vi "strip returns.vi"(8 "error in (no error)":errorcluster, 11 "Language data":T1) -> (0 "error out":errorcluster, 3 "Language data out":T1)   [LabVIEW 2015, in "AguaClara Library.lvlib"]
uses:
  AguaClara Library.lvlib
  Variable cluster.ctl
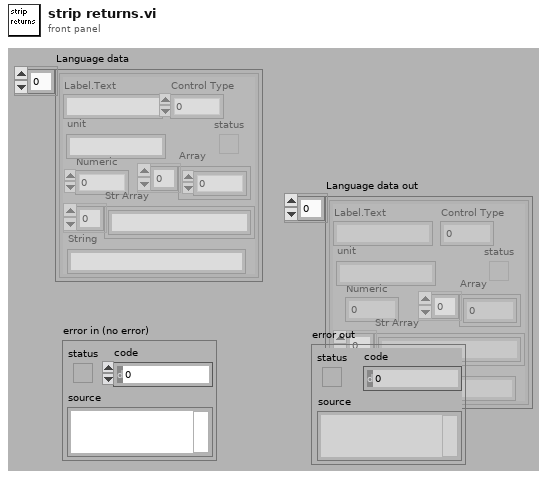
[diagram p1: front panel]
types:
  T1 = typedef "Variable cluster.ctl" = cluster{"Label.Text":string, "Control Type":u32, "Numeric":dbl, "Array":dbl[], "status":bool, "Str Array":string[], "String":string, "unit":string}[]
  T2 = cluster{"Label.Text":string, "Control Type":u32, "Numeric":dbl, "Array":dbl[], "status":bool, "Str Array":string[], "String":string, "unit":string}
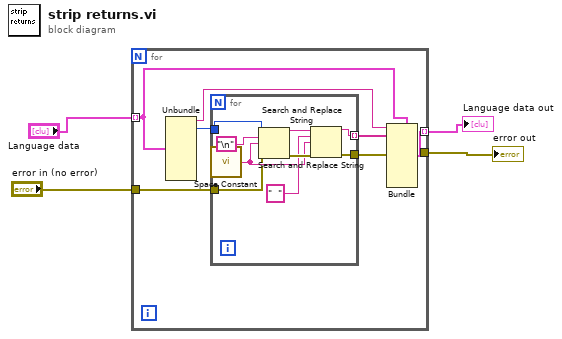
[diagram p0: block diagram]
diagram:
  n1 = for {
    tunnel: "Language data" -> [w10] mode=indexing
    tunnel: [w7] -> w3 mode=indexing
    tunnel: "error in (no error)" -> [w6]
    tunnel: [w5] -> w1
    n2 = Unbundle(w10) -> ("Label.Text"=w9:string, "Control Type"=w11:u32)  [unwired: 6 out]
    n3 = for {
      tunnel: w11 -> [w20]
      tunnel: [w15] -> w8 mode=indexing
      tunnel: w6 -> [w14]
      tunnel: [w13] -> w5
      n4 = call <vilib>:"Space Constant.vi"() -> ("String"=w16:string)
      n5 = Search and Replace String(input string=w20, search string="\n", replace string=w16, error in=w14) -> (result string=w19:string, error out=w18:errorcluster)  [unwired: 4 in, 2 out]
      n6 = Search and Replace String(input string=w19, search string="  ", replace string=w16, error in=w18) -> (result string=w15:string, error out=w13:errorcluster)  [unwired: 4 in, 2 out]
    }
    n7 = Bundle(cluster=w10, "Label.Text"=w9, "Control Type"=w8) -> (w7:T2)  [unwired: 6 in]
  }
  "Language data out" <- w3
  "error out" <- w1
